vi "UNITTEST-JSON-RPC-cluster.vi"(8 "error in (no error)":errorcluster) -> (0 "error out":errorcluster)   [LabVIEW 2019]
uses:
  <vilib>/numeric/Random Number (Range) DBL.vi
  <vilib>/numeric/Random Number (Range) U64.vi
  4c12f335-3af6-49f5-9257-0130b4f6318c.vi
  e861ad0b-bed5-4796-b07d-8449c8f87c08.vi
  <vilib>/numeric/sub_Random U32.vi
  4c12f335-3af6-49f5-9257-0130b4f6318c.vi/7b8b0f69-2f54-4be0-9abe-caa8645179b0.vi
  4c12f335-3af6-49f5-9257-0130b4f6318c.vi/307d6119-f25b-468d-b3e0-ef9f1a1a6fd2.vi
  e861ad0b-bed5-4796-b07d-8449c8f87c08.vi/dab2e044-56e2-4a2a-97c6-8deb14d6665e.vi
  e861ad0b-bed5-4796-b07d-8449c8f87c08.vi/55732a74-c736-46f3-938e-d0df42ffec67.vi
  <vilib>/Utility/Data Type/Get Type Information.vi
  <vilib>/JDP Science/JSONtext/JSON text to Variant.vi
  <vilib>/addons/_JKI Toolkits/Caraya/classes/Assert/Assert Almost Equal_Float.vi
  <vilib>/addons/_JKI Toolkits/Caraya/classes/Assert/Assert Equal Value_Variant.vi
  <vilib>/addons/_JKI Toolkits/Caraya/classes/Assert/Assert Not Error.vi
  <vilib>/JDP Science/JSONtext/LVClass Serializer/JSONtext LVClass Serializer.lvclass
  JSON-RPC/JSON-RPC.lvlib
  <vilib>/addons/_JKI Toolkits/Caraya/classes/Assert/Assert.lvclass
  <vilib>/addons/_JKI Toolkits/Caraya/classes/Test/Test.lvclass
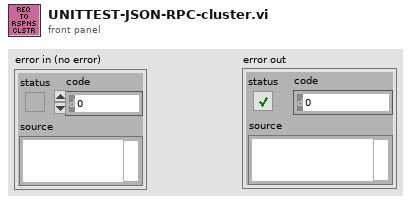
[diagram p1: front panel]
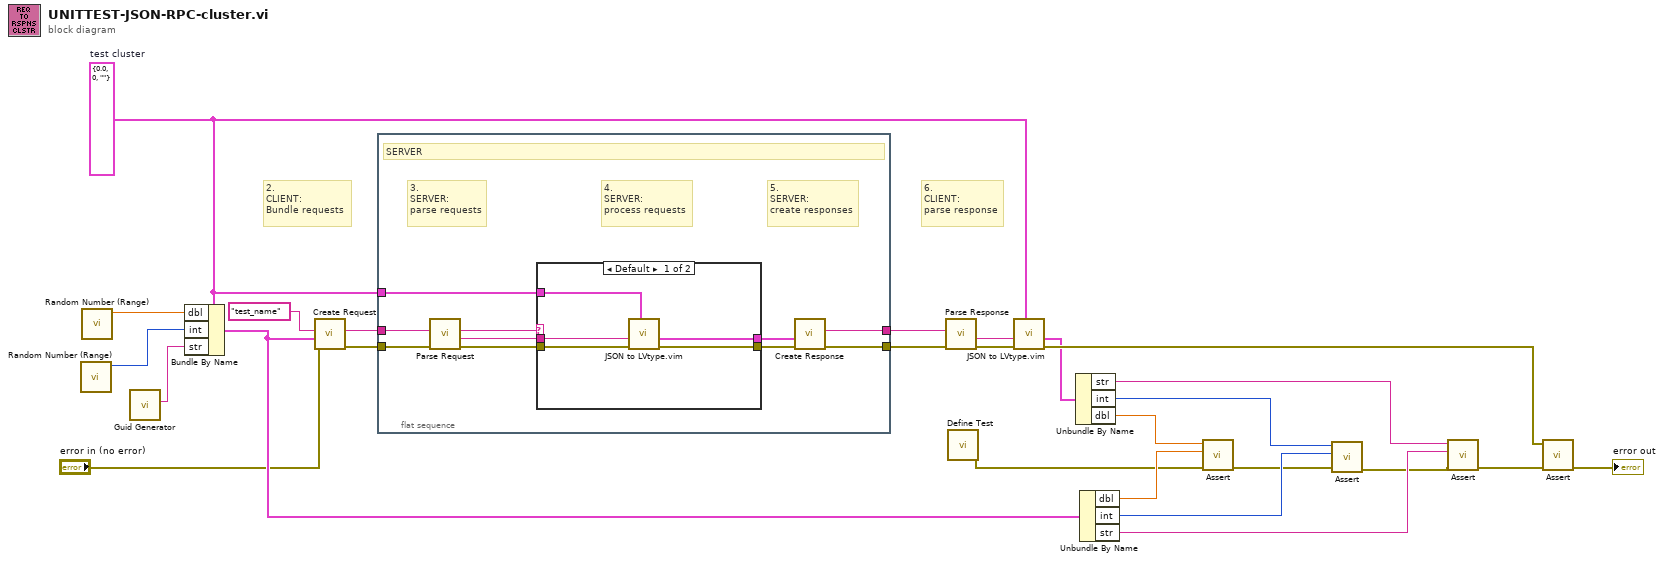
[diagram p0: block diagram]
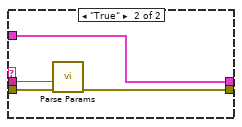
[diagram p2: hidden frame]
diagram:
  w18 = cluster{"dbl":dbl, "int":i32, "str":string} {"dbl"=0.0, "int"=0, "str"=""}  # test cluster
  # "6.\nCLIENT:\nparse response"
  # "2.\nCLIENT:\nBundle requests"
  n1 = call-poly <vilib>:"Random Number (Range).vi"() -> ("number"=w22:u64)  [unwired: 11 in]
  n2 = call-poly <vilib>:"Random Number (Range).vi"() -> ("number"=w21:dbl)  [unwired: 11 in]
  n3 = call <vilib>:"Guid Generator.vi"() -> ("GUID"=w20:string)  [unwired: 10 in, 1 out]
  n4 = Bundle By Name(cluster=w18, "dbl"=w21, "int"=w22, "str"=w20) -> (w4:cluster{"dbl":dbl, "int":i32, "str":string})
  n5 = call "Create Request.vi"("error in (no error)"="error in (no error)", "params"=w4, "method"="test_name") -> ("error out"=w25:errorcluster, "<JSON> Requests"=w26:string)  [unwired: 6 in, 1 out]
  n6 = flat-sequence {
    tunnel: w26 -> [w36]
    tunnel: w25 -> [w32]
    tunnel: [w31] -> w24
    tunnel: [w30] -> w23
    tunnel: w18 -> [w28]
    frame #0 {
      # "3.\nSERVER:\nparse requests"
      # "4.\nSERVER:\nprocess requests"
      # "5.\nSERVER:\ncreate responses"
      # "SERVER"
      n7 = call "Parse Request.vi"("error in (no error)"=w32, "<JSON> Requests"=w36) -> ("error out"=w33:errorcluster, "Params"=w34:string, "Methods"=w35:string)  [unwired: 6 in, 1 out]
      n8 = case shown="Default" w35 {
        tunnel: w34 -> [w38 w45]
        tunnel: w33 -> [w41 w44]
        tunnel: [w40 w43] -> w29
        tunnel: w28 -> [w39 w42]
        tunnel: [w37 w42] -> w27
        frame Default {
          n9 = call "JSON to LVtype.vim"("type"=w39, "error in (no error)"=w41, "JSON Data in"=w38) -> ("error out"=w40:errorcluster, "Data out"=w37:cluster{"dbl":dbl, "int":i32, "str":string})  [unwired: 7 in]
        }
        frame "True" {
          n10 = call "Parse Params.vi"("error in (no error)"=w44, "<JSON> Params"=w45) -> ("error out"=w43:errorcluster)  [unwired: 7 in, 2 out]
        }
      }
      n11 = call "Create Response.vi"("error in (no error)"=w29, "result"=w27) -> ("error out"=w30:errorcluster, "<JSON> Response"=w31:string)  [unwired: 8 in]
    }
  }
  n12 = call "Parse Response.vi"("error in (no error)"=w23, "<JSON> Response"=w24) -> ("error out"=w19:errorcluster, "results"=w2:string)  [unwired: 7 in, 1 out]
  n13 = call <vilib>:"Define Test.vi"() -> ("error out"=w6:errorcluster)  [unwired: 10 in, 1 out]
  n14 = call "JSON to LVtype.vim"("type"=w18, "error in (no error)"=w19, "JSON Data in"=w2) -> ("error out"=w9:errorcluster, "Data out"=w1:cluster{"dbl":dbl, "int":i32, "str":string})  [unwired: 7 in]
  n15 = Unbundle By Name(w1) -> ("str"=w14:string, "int"=w15:i32, "dbl"=w17:dbl)
  n16 = Unbundle By Name(w4) -> ("dbl"=w16:dbl, "int"=w13:i32, "str"=w11:string)
  n17 = call-poly <vilib>:"Assert.vi"("error in (no error)"=w6, "Y"=w16, "X"=w17) -> ("error out"=w12:errorcluster)  [unwired: 7 in, 1 out]
  n18 = call-poly <vilib>:"Assert.vi"("error in (no error)"=w12, "Y"=w13, "X"=w15) -> ("error out"=w10:errorcluster)  [unwired: 7 in, 1 out]
  n19 = call-poly <vilib>:"Assert.vi"("error in (no error)"=w10, "Y"=w11, "X"=w14) -> ("error out"=w8:errorcluster)  [unwired: 7 in, 1 out]
  n20 = call-poly <vilib>:"Assert.vi"("error in (no error)"=w8, "Not Error?"=w9) -> ("error out"=→"error out":errorcluster)  [unwired: 8 in, 1 out]
